vi "Unique Elements.vi"(1 "P-waves":dbl[](array[numeric]) format="%.2p") -> (0 "Unique P-Waves":dbl[](array[numeric]))   [LabVIEW 2018]
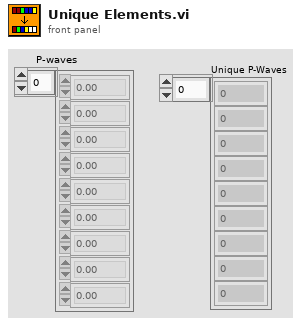
[diagram p1: front panel]
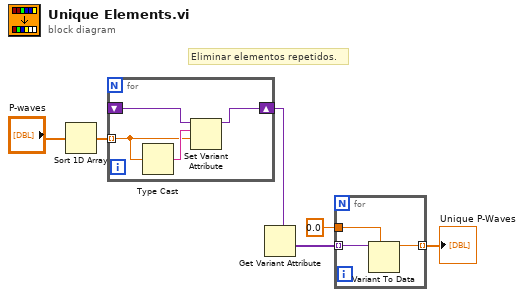
[diagram p0: block diagram]
diagram:
  # "Eliminar elementos repetidos."
  n1 = Sort 1D Array(array="P-waves") -> (sorted array=w3:dbl[])
  n2 = for {
    shift-right: [w9] -> w4
    shift-left: _ -> [w10]
    tunnel: w3 -> [w7] mode=indexing
    n3 = Type Cast(x=w7) -> (*(type *) &x=w8:string)  [unwired: 1 in]
    n4 = Set Variant Attribute(Variant=w10, name=w8, value=w7) -> (Variant out=w9:variant)  [unwired: 1 in, 2 out]
  }
  n5 = Get Variant Attribute(Variant=w4) -> (values=w5:variant[])  [unwired: 3 in, 3 out]
  n6 = for {
    tunnel: w5 -> [w13] mode=indexing
    tunnel: 0.0 -> [w12]
    tunnel: [w11] -> w6 mode=indexing
    n7 = Variant To Data(type=w12, Variant=w13) -> (data=w11:dbl)  [unwired: 1 in, 1 out]
  }
  "Unique P-Waves" <- w6
